vi "SetComparison.vi"(8 "error in":errorcluster, 10 "Comparison":bool, 11 "BooleanMeasureLimit in":refnum<class "BooleanMeasureLimit.lvclass">) -> (0 "error out":errorcluster, 3 "BooleanMeasureLimit out":refnum<class "BooleanMeasureLimit.lvclass">)   [LabVIEW 2021, in "ProligentXMLGenerator.lvlib" / "BooleanMeasureLimit.lvclass"]
doc: "Boolean Measure Limit Comparison"
uses:
  BooleanMeasureLimit.lvclass
  BooleanMeasureLimit.lvclass/BooleanMeasureLimit.ctl
  Base/Boolean/Boolean.lvclass
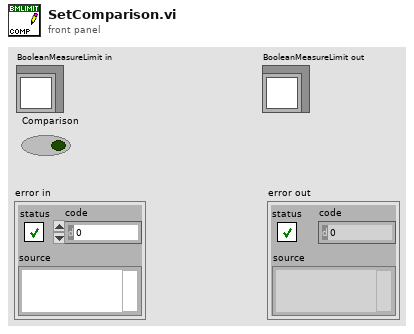
[diagram p1: front panel]
types:
  T1 = typedef "ProligentXMLGenerator.lvlib/BooleanMeasureLimit.lvclass/Data.ctl" = cluster{"Comparison":refnum<class "Boolean.lvclass">}
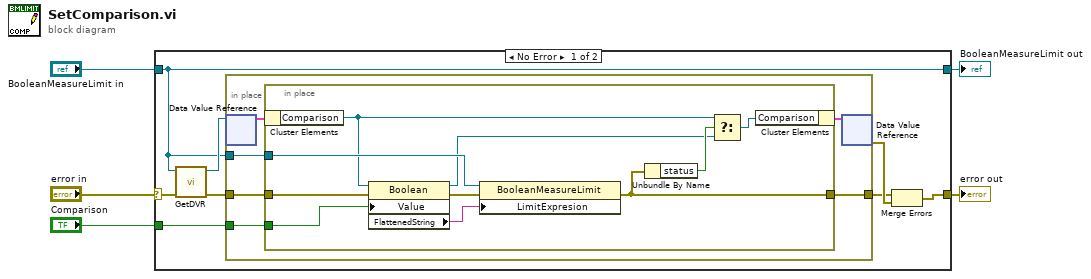
[diagram p0: block diagram]
diagram:
  n1 = case shown="No Error" "error in" {
    selector: "error in" -> [w7 w30]
    tunnel: "BooleanMeasureLimit in" -> [w6 w31]
    tunnel: [w12 w30] -> w3
    tunnel: "Comparison" -> [w11 _]
    tunnel: [w6 w31] -> w1
    frame No Error {
      n2 = call "GetDVR.vi"("error in"=w7, "BooleanMeasureLimit"=w6) -> ("error out"=w10:errorcluster, "DVRReference"=w13:refnum<data-value>)  [unwired: 8 in]
      n3 = in-place "In Place Element Structure" {
        in-place-border: w11 -> [w19]
        in-place-border: w10 -> [w16]
        in-place-border: [w15] -> w8
        in-place-border: w6 -> [w14]
        n4 = in-place-dvr #1(w13) -> (w18:T1)  [unwired: 1 out]
        n5 = in-place "In Place Element Structure" {
          in-place-border: w19 -> [w28]
          in-place-border: w16 -> [w27]
          in-place-border: [w22] -> w15
          in-place-border: w14 -> [w29]
          n6 = in-place-cluster #2(w18) -> ("Comparison"=w24:refnum<class "Boolean.lvclass">)
          n7 = property class="Boolean"(reference=w24, error in=w27, "Value"=w28) -> (reference out=w20:refnum<class "Boolean.lvclass">, error out=w25:errorcluster, "FlattenedString"=w26:string)
          n8 = property class="BooleanMeasureLimit"(reference=w29, error in=w25, "LimitExpresion"=w26) -> (error out=w22:errorcluster)  [unwired: 1 out]
          n9 = Unbundle By Name(w22) -> ("status"=w21:bool)
          n10 = Select(t=w24, s=w21, f=w20) -> (s? t:f=w23:refnum<class "Boolean.lvclass">)
          n11 = in-place-cluster #2("Comparison"=w23) -> (w17:T1)
        }
        n12 = in-place-dvr #1(w17) -> (w9:errorcluster)  [unwired: 1 out]
      }
      n13 = Merge Errors(w8, w9) -> (w12:errorcluster)
    }
    frame Error {
    }
  }
  "error out" <- w3
  "BooleanMeasureLimit out" <- w1
